vi "DispenserPatternRotate.vi"(0 "VISA resource name":refnum<visa-resource-name>="COM6", 1 "X":dbl=435.404 format="%#_13g", 2 "AngleInDeg":dbl=90.0 format="%#_13g", 3 "Y":dbl=905.746 format="%#_13g", 5 "Serial Configuration":T1={"Baud Rate "=115200, "Parity "=0, "Data Bits "=8, "Stop Bits"=10} {"Stop Bits" items=["1.0"=10, "1.5"=15, "2.0"=20]; "Data Bits" items=["7"=7, "8"=8]; "Parity" items=["None", "Odd", "Even"]; "Baud Rate" items=["9600"=9600, "19200"=19200, "38400"=38400, "115200"=115200]}, 7 "controller in":refnum<k24>, 9 "Path":path=path "C:/Users/TTUHEP/Documents/LabVIEW/Data/Patterns/PCB_base_Dec21_Combined.ngc", 11 "Pressure":dbl[](array[numeric])=[27.0, 27.0, 27.0, 27.0], 12 "Z":dbl=71.609 format="%#_13g", 13 "error in (no error)":errorcluster) -> (4 "Comm":string, 6 "Speed":dbl format="%#_13g", 8 "controller out":refnum<k24>, 10 "Time(ms)":dbl, 15 "error out":errorcluster)   [LabVIEW 2019]
uses:
  C:/Users/TTUHEP/Documents/LabVIEW/Other Models/2010/Bin/Aerotech.A3200.dll
  Other Models/2010/Bin/Aerotech.A3200.dll
  <vilib>/Utility/file.llb/Read Delimited Spreadsheet (string).vi
  Other Models/EFD Ultimus V/EFD Ultimus V.lvlib
panel:
  in  "file path (use dialog) 2":path
  in  "file path (use dialog)":path
  # "Origin"
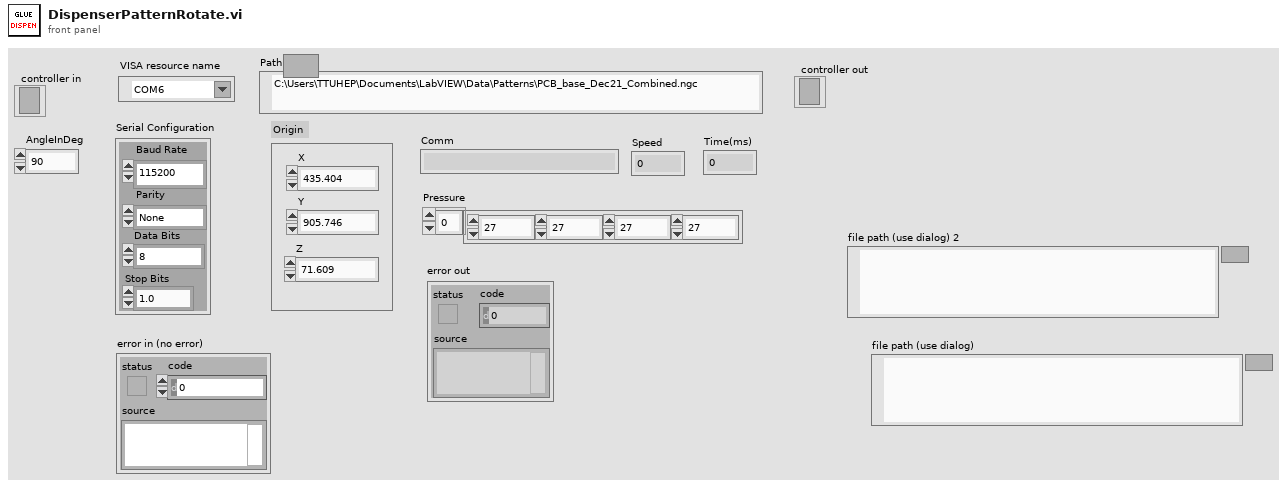
[diagram p1: front panel]
types:
  T1 = cluster{"Baud Rate ":u32, "Parity ":u16, "Data Bits ":u16, "Stop Bits":u16}
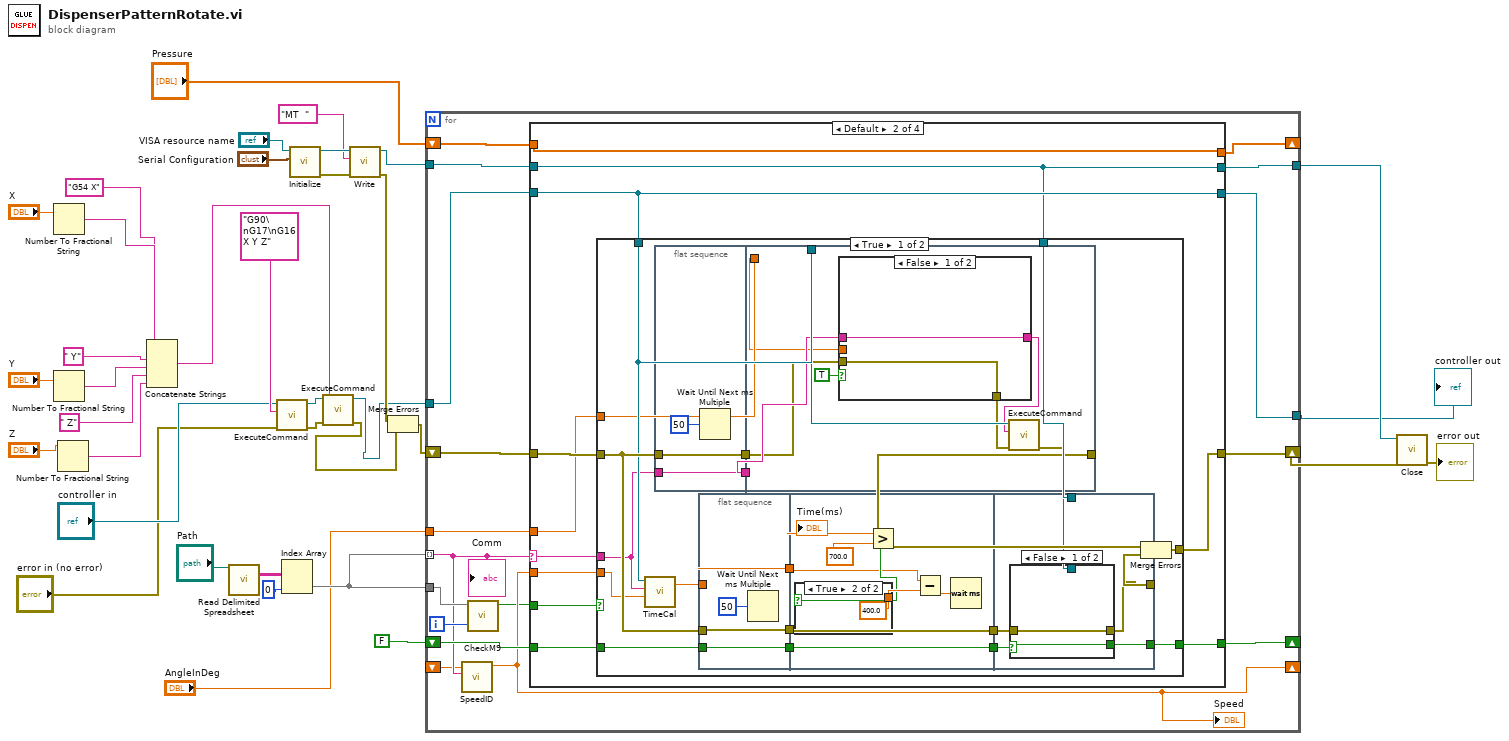
[diagram p0: block diagram]
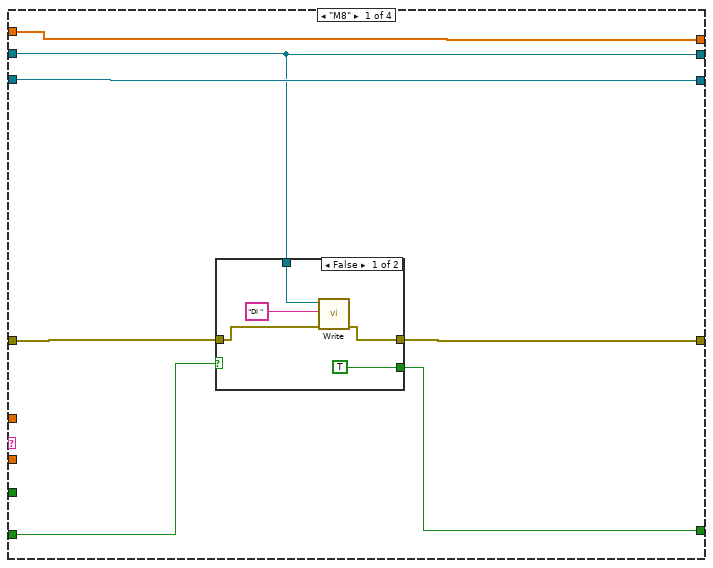
[diagram p2: hidden frame]
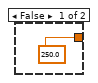
[diagram p4: hidden frame]
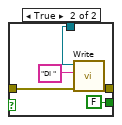
[diagram p5: hidden frame]
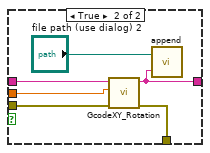
[diagram p6: hidden frame]
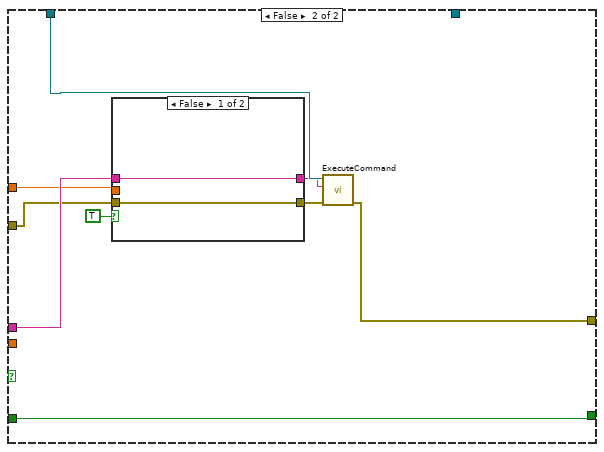
[diagram p7: hidden frame]
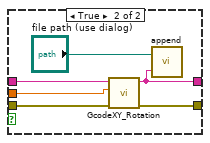
[diagram p8: hidden frame]
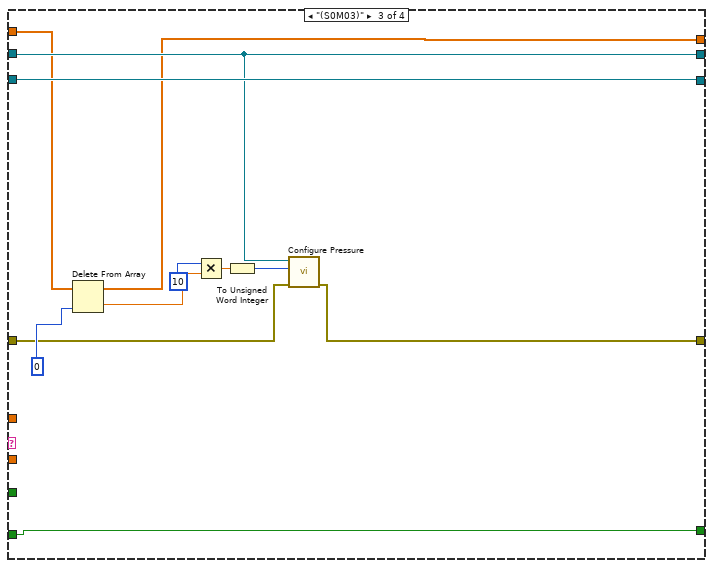
[diagram p9: hidden frame]
diagram:
  n1 = Number To Fractional String(number="X") -> (F-format string=w21:string)  [unwired: 3 in]
  n2 = Number To Fractional String(number="Y") -> (F-format string=w23:string)  [unwired: 3 in]
  n3 = Number To Fractional String(number="Z") -> (F-format string=w25:string)  [unwired: 3 in]
  n4 = Concatenate Strings("G54 X", w21, " Y", w23, " Z", w25) -> (w19:string)
  n5 = call-poly <vilib>:"Read Delimited Spreadsheet.vi"("file path (dialog if empty)"="Path") -> ("all rows"=w35:string[][])  [unwired: 9 in, 5 out]
  n6 = call "ExecuteCommand.vi"("error in (no error)"="error in (no error)", "Command Code"="G90\nG17\nG16 X Y Z", "controller in"="controller in") -> ("error out"=w7:errorcluster, "controller out"=w10:refnum<k24>)  [unwired: 6 in, 1 out]
  n7 = Index Array(array=w35, index (col)=0) -> (element=w12:string[])  [unwired: 1 in]
  n8 = call "Initialize.vi"("Serial Configuration"="Serial Configuration", "VISA resource name"="VISA resource name") -> ("error out"=w16:errorcluster, "VISA resource name out"=w15:refnum<visa-resource-name>)  [unwired: 8 in]
  n9 = call "ExecuteCommand.vi"("error in (no error)"=w7, "Command Code"=w19, "controller in"=w10) -> ("error out"=w1:errorcluster, "controller out"=w2:refnum<k24>)  [unwired: 6 in, 1 out]
  n10 = call "Write.vi"("error in (no error)"=w16, "Command To Write"="MT  ", "VISA resource name"=w15) -> ("error out"=w13:errorcluster, "VISA resource name out"=w17:refnum<visa-resource-name>)  [unwired: 7 in]
  n11 = Merge Errors(w13, w1) -> (w30:errorcluster)
  n12 = for {
    tunnel: w12 -> [w44] mode=indexing
    shift-right: [w41] -> w5
    shift-left: w30 -> [w49]
    shift-right: [w51] -> _
    shift-left: FALSE -> [w52]
    tunnel: w2 -> [w50]
    tunnel: [w53] -> w11
    tunnel: w17 -> [w48]
    tunnel: [w47] -> w29
    tunnel: w12 -> [w46]
    shift-right: [w42] -> _
    shift-left: _ -> [w43]
    shift-right: [w39] -> _
    shift-left: "Pressure" -> [w40]
    tunnel: "AngleInDeg" -> [w38]
    i -> [w45]
    n13 = call "SpeedID.vi"("String"=w44, "Speed In"=w43) -> ("Speed Out"=w42:dbl)  [unwired: 9 in]
    "Speed" <- w42
    n14 = call "CheckM9.vi"("Index"=w45, "Comm list"=w46) -> ("Gonna Stop Next"=w37:bool)  [unwired: 9 in]
    n15 = case shown="Default" w44 {
      selector: w44 -> [_ w76 _ _]
      tunnel: w49 -> [w55 w78 w160 w174]
      tunnel: w50 -> [w60 w77 w170 w172]
      tunnel: [w59 w70 w159 w174] -> w41
      tunnel: [w60 w77 w170 w172] -> w53
      tunnel: w52 -> [w58 w74 w169 w175]
      tunnel: [w57 w73 w169 w175] -> w51
      tunnel: w48 -> [w56 w75 w168 w173]
      tunnel: [w56 w75 w168 w173] -> w47
      tunnel: w37 -> [_ w72 _ _]
      tunnel: w42 -> [_ w71 _ _]
      tunnel: w40 -> [w54 w69 w166 w171]
      tunnel: [w54 w69 w164 w171] -> w39
      tunnel: w38 -> [_ w68 _ _]
      frame "M8" {
        n16 = case shown="False" w58 {
          selector: w58 -> [_ w66]
          tunnel: w55 -> [w63 w67]
          tunnel: [w62 w67] -> w59
          tunnel: [TRUE w66] -> w57
          tunnel: w56 -> [w64 _]
          frame False {
            n17 = call "Write.vi"("error in (no error)"=w63, "Command To Write"="DI ", "VISA resource name"=w64) -> ("error out"=w62:errorcluster)  [unwired: 7 in, 1 out]
          }
          frame True {
          }
        }
      }
      frame Default {
        n18 = case shown="True" w72 {
          tunnel: w78 -> [w89 w146]
          tunnel: [w87 w150] -> w70
          tunnel: w77 -> [w82 w149]
          tunnel: w76 -> [w81 w147]
          tunnel: w75 -> [w95 _]
          tunnel: w74 -> [w97 w148]
          tunnel: [w96 w148] -> w73
          tunnel: w71 -> [w80 _]
          tunnel: w68 -> [w79 w143]
          frame True {
            n19 = call "TimeCal.vi"("Speed In"=w80, "Command"=w81, "controller in"=w82) -> ("Time(ms)"=w83:dbl)  [unwired: 7 in, 1 out]
            n20 = flat-sequence {
              tunnel: w81 -> [w124]
              tunnel: [w124] -> w90
              tunnel: w89 -> [w123]
              tunnel: [w123] -> w88
              tunnel: w90 -> [w129]
              tunnel: w88 -> [w127]
              tunnel: [w133] -> w85
              tunnel: w82 -> [w132]
              tunnel: w79 -> [w128]
              frame #0 {
                n21 = Wait Until Next ms Multiple(millisecond multiple=50) -> ()  [unwired: 1 out]
              }
              frame #1 {
                n22 = case shown="False" TRUE {
                  tunnel: w129 -> [w135 w141]
                  tunnel: w127 -> [w134 w140]
                  tunnel: [w135 w138] -> w130
                  tunnel: w128 -> [_ w139]
                  tunnel: [w134 w136] -> w126
                  frame False {
                  }
                  frame True {
                    n23 = call "GcodeXY_Rotation.vi"("error in"=w140, "AngleInDeg"=w139, "GCodeIn"=w141) -> ("error out 2"=w136:errorcluster, "GCodeOut"=w138:string)  [unwired: 3 in]
                    n24 = call "append.vi"("text"=w138, "file path (use dialog)"="file path (use dialog) 2") -> ()  [unwired: 1 out]
                  }
                }
                n25 = call "ExecuteCommand.vi"("error in (no error)"=w126, "Command Code"=w130, "controller in"=w132) -> ("error out"=w133:errorcluster)  [unwired: 6 in, 2 out]
              }
            }
            n26 = flat-sequence {
              tunnel: w97 -> [w101]
              tunnel: [w101] -> w93
              tunnel: [w99] -> w92
              tunnel: w89 -> [w99]
              tunnel: w83 -> [w98]
              tunnel: [w98] -> w84
              tunnel: [w108] -> w94
              tunnel: w93 -> [w108]
              tunnel: w92 -> [w107]
              tunnel: [w107] -> w91
              tunnel: w84 -> [w102]
              tunnel: [w114] -> w96
              tunnel: [w113] -> w86
              tunnel: w95 -> [w112]
              tunnel: w94 -> [w115]
              tunnel: w91 -> [w111]
              frame #0 {
                n27 = Wait Until Next ms Multiple(millisecond multiple=50) -> ()  [unwired: 1 out]
              }
              frame #1 {
                n28 = Greater?(x=w102, y=700.0) -> (0:w104:bool)
                n29 = case shown="True" w104 {
                  tunnel: [250.0 400.0] -> w105
                  frame False {
                  }
                  frame True {
                  }
                }
                n30 = Subtract(x=w102, y=w105) -> (x-y=w106:dbl)
                n31 = Wait (ms)(milliseconds to wait=w106) -> ()  [unwired: 1 out]
                "Time(ms)" <- w102
              }
              frame #2 {
                n32 = case shown="False" w115 {
                  selector: w115 -> [w116 _]
                  tunnel: w111 -> [w117 w121]
                  tunnel: [w117 w120] -> w113
                  tunnel: [w116 FALSE] -> w114
                  tunnel: w112 -> [_ w119]
                  frame False {
                  }
                  frame True {
                    n33 = call "Write.vi"("error in (no error)"=w121, "Command To Write"="DI ", "VISA resource name"=w119) -> ("error out"=w120:errorcluster)  [unwired: 7 in, 1 out]
                  }
                }
              }
            }
            n34 = Merge Errors(w85, w86) -> (w87:errorcluster)
          }
          frame False {
            n35 = case shown="False" TRUE {
              tunnel: w147 -> [w152 w158]
              tunnel: w146 -> [w151 w157]
              tunnel: [w151 w156] -> w145
              tunnel: [w152 w154] -> w144
              tunnel: w143 -> [_ w155]
              frame False {
              }
              frame True {
                n36 = call "GcodeXY_Rotation.vi"("error in"=w157, "AngleInDeg"=w155, "GCodeIn"=w158) -> ("error out 2"=w156:errorcluster, "GCodeOut"=w154:string)  [unwired: 3 in]
                n37 = call "append.vi"("text"=w154, "file path (use dialog)"="file path (use dialog)") -> ()  [unwired: 1 out]
              }
            }
            n38 = call "ExecuteCommand.vi"("error in (no error)"=w145, "Command Code"=w144, "controller in"=w149) -> ("error out"=w150:errorcluster)  [unwired: 6 in, 2 out]
          }
        }
      }
      frame "(S0M03)" {
        n39 = Delete From Array(array=w166, index=0) -> (deleted portion=w163:dbl, array with subset deleted=w164:dbl[])  [unwired: 1 in]
        n40 = Multiply(x=10, y=w163) -> (x*y=w162:dbl)
        n41 = To Unsigned Word Integer(number=w162) -> (unsigned 16bit integer=w161:u16)
        n42 = call "Configure Pressure.vi"("error in (no error)"=w160, "Pressure Setting (0000)"=w161, "VISA resource name"=w168) -> ("error out"=w159:errorcluster)  [unwired: 7 in, 1 out]
      }
      frame "M9" {
      }
    }
    "Comm" <- w44
  }
  "controller out" <- w11
  n43 = call "Close.vi"("error in (no error)"=w5, "VISA resource name"=w29) -> ("error out"=→"error out":errorcluster)  [unwired: 9 in]
